vi "Exemple_Metrics_Pairwise_Paired_Distances.vi"() -> ()   [LabVIEW 2020]
uses:
  Objet/6 - Datasets Transformation/6.8 - Pairwise metrics, Affinities and Kernels/Paired_distances/Paired_distances.vi
panel:
  in  "paired_distances":cluster{"metric":string}={"metric"="euclidean"}
  in  "error in":errorcluster caption="entrée d'erreur"
  in  "Y":string[][](array[string])=[["1", "2"], ["0", "3"]]
  in  "X":string[][](array[string])=[["1", "2"], ["3", "4"]]
  out "Data":T1
  out "error out":errorcluster caption="sortie d'erreur"
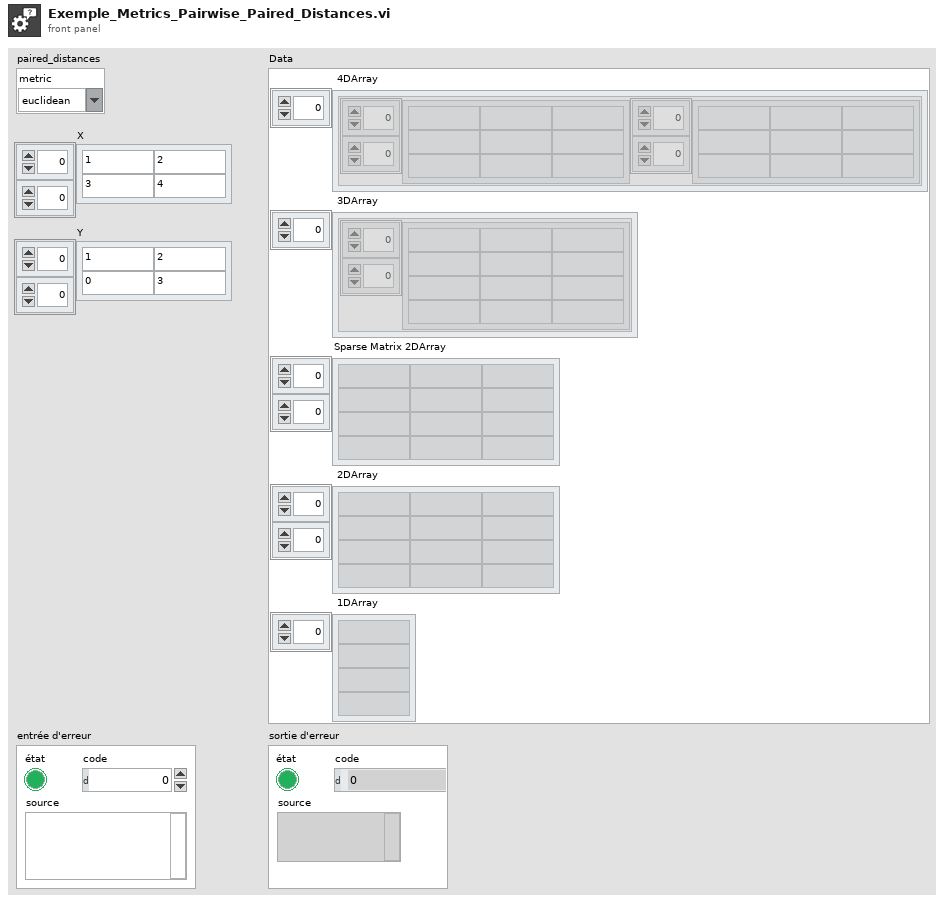
[diagram p1: front panel]
types:
  T1 = cluster{" 4DArray":cluster{"1":string[][], "2":string[][]}[], " 3DArray":cluster{"Tableau":string[][]}[], "Sparse Matrix 2DArray":string[][], " 2DArray":string[][], " 1DArray":string[]}
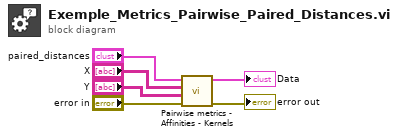
[diagram p0: block diagram]
diagram:
  n1 = call-poly "Pairwise metrics - Affinities - Kernels.vi"("error in"="error in", "Y"="Y", "X"="X", "paired_distances"="paired_distances") -> ("error out"=→"error out":errorcluster, "Data"=→"Data":T1)  [unwired: 6 in]
